vi "ECDChromBetrachterPC.vi"() -> ()   [LabVIEW 2010]
panel:
  in  "Zyklus":i32 min=0 max=385 step=1
  in  "Methode":i32 min=0 max=0 step=1
  out "Name":string
  in  "Beenden":bool
  out "Chrom":cluster{dbl, dbl}[](graph)
  in  "anzeigen":bool
  in  "Pfad":path
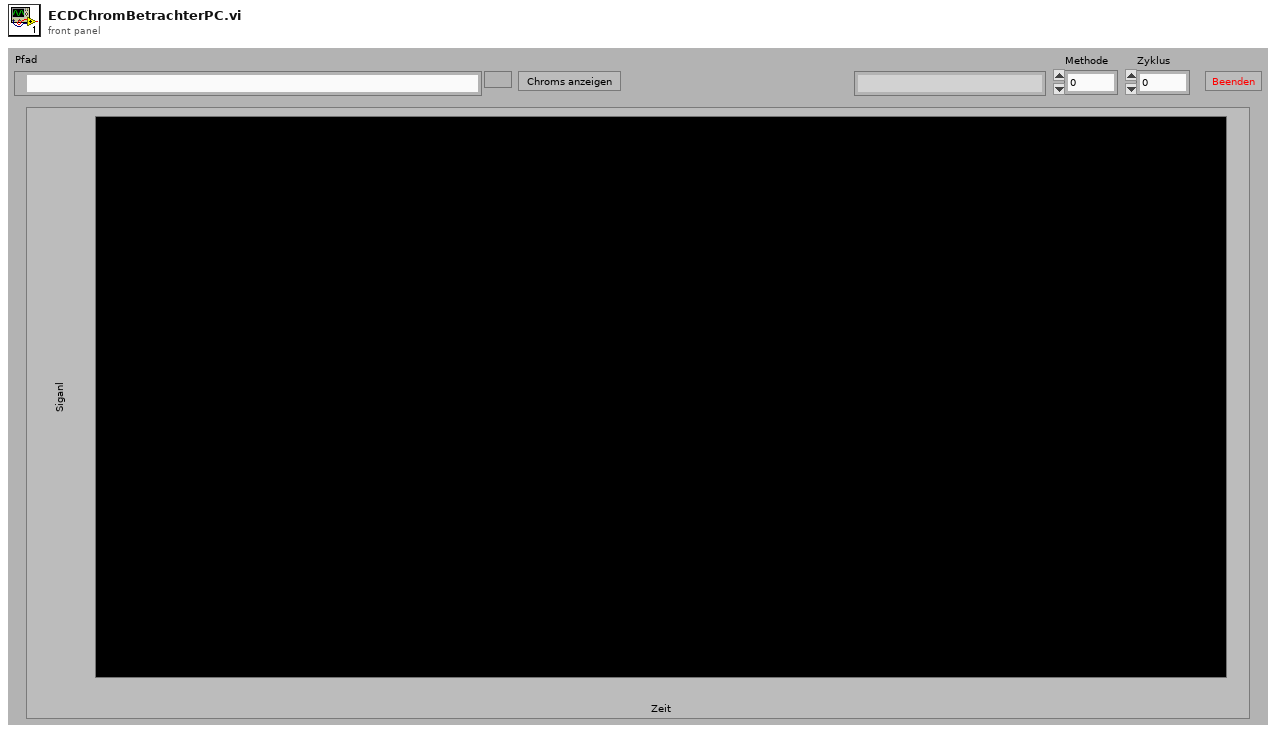
[diagram p1: front panel]
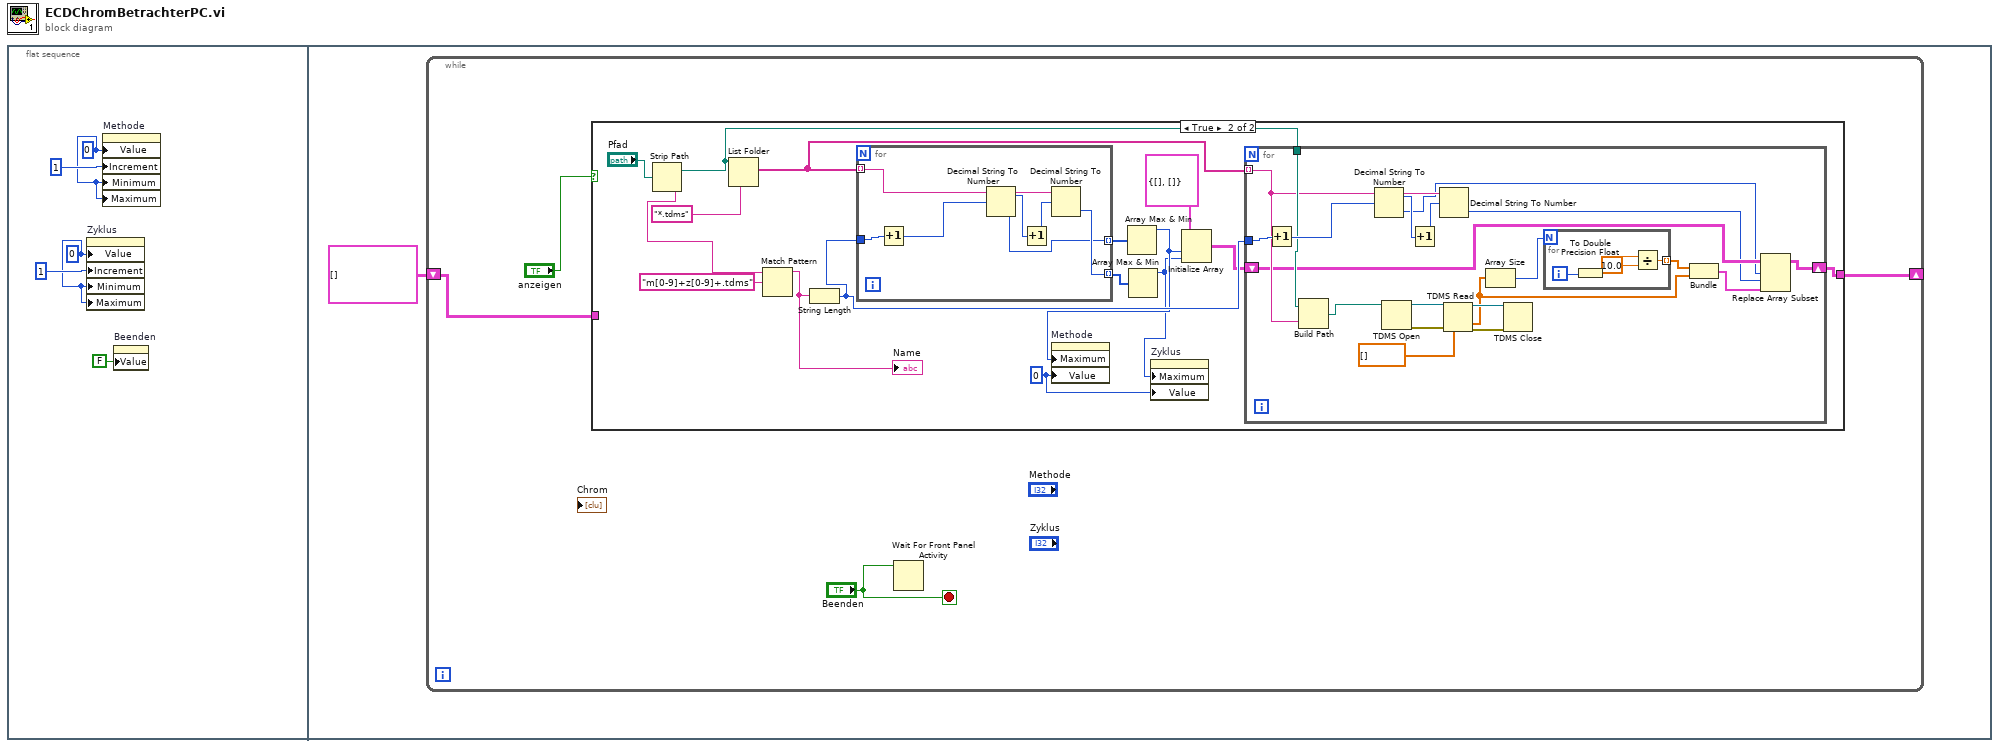
[diagram p0: block diagram]
diagram:
  n1 = flat-sequence {
    frame #0 {
      w2 = 0 ("Methode")
      w4 = 0 ("Methode")
      n2 = property on="Zyklus" class="DigWert (strikt)"("Value"=w2, "Increment"=1, "Minimum"=w2, "Maximum"=w2) -> ()  [unwired: 2 in, 2 out]
      n3 = property on="Methode" class="DigWert (strikt)"("Value"=w4, "Increment"=1, "Minimum"=w4, "Maximum"=w4) -> ()  [unwired: 2 in, 2 out]
      n4 = property on="Beenden" class="Bool. (strikt)"("Value"=FALSE ("Beenden")) -> ()  [unwired: 2 in, 2 out]
    }
    frame #1 {
      n5 = while {
        shift-right: [w8] -> _
        shift-left: cluster{dbl[], dbl[]}[][] [] -> [w7]
        stop <- "Beenden" stop-if-true
        n6 = case shown="True" "anzeigen" {
          tunnel: [w11 w15] -> w8
          tunnel: w7 -> [w11 _]
          frame False {
          }
          frame True {
            w12 = 0 ("Methode")
            n7 = Strip Path(path="Pfad") -> (stripped path=w17:path, name=w25:string)
            n8 = List Folder(path=w17, pattern="*.tdms" ("Muster")) -> (filenames=w18:string[])  [unwired: 2 in, 3 out]
            n9 = Match Pattern(string=w25, regular expression="m[0-9]+z[0-9]+.tdms" ("Regulärer Ausdruck")) -> (before substring=w23:string)  [unwired: 1 in, 3 out]
            "Name" <- w23
            n10 = String Length(string=w23) -> (length=w19:i32)
            n11 = for {
              tunnel: w18 -> [w54] mode=indexing
              tunnel: w19 -> [w56]
              tunnel: [w53] -> w21 mode=indexing
              tunnel: [w52] -> w22 mode=indexing
              n12 = Increment(x=w56) -> (x+1=w55:i32)
              n13 = Decimal String To Number(string=w54, offset=w55) -> (offset past number=w58:i32, number=w52:i32)  [unwired: 1 in]
              n14 = Increment(x=w58) -> (x+1=w57:i32)
              n15 = Decimal String To Number(string=w54, offset=w57) -> (number=w53:i32)  [unwired: 1 in, 1 out]
            }
            n16 = Array Max & Min(array=w22) -> (max value=w14:i32)  [unwired: 3 out]
            n17 = property on="Methode" class="DigWert (strikt)"("Maximum"=w14, "Value"=w12) -> ()  [unwired: 2 in, 2 out]
            n18 = Array Max & Min(array=w21) -> (max value=w13:i32)  [unwired: 3 out]
            n19 = property on="Zyklus" class="DigWert (strikt)"("Maximum"=w13, "Value"=w12) -> ()  [unwired: 2 in, 2 out]
            n20 = Initialize Array(cluster{dbl[], dbl[]} {[], []} ("Ausgangs-Cluster"), w14, w13) -> (w16:cluster{dbl[], dbl[]}[][])
            n21 = for {
              tunnel: w18 -> [w36] mode=indexing
              tunnel: w19 -> [w45]
              tunnel: w17 -> [w37]
              shift-right: [w28] -> w15
              shift-left: w16 -> [w32]
              n22 = Increment(x=w45) -> (x+1=w44:i32)
              n23 = Build Path(base path=w37, name or relative path=w36) -> (appended path=w43:path)
              n24 = Decimal String To Number(string=w36, offset=w44) -> (offset past number=w47:i32, number=w31:i32)  [unwired: 1 in]
              n25 = TDMS Open(11:w43) -> (0:w41:errorcluster, 3:w42:refnum<k34>)  [unwired: 5 in]
              n26 = Increment(x=w47) -> (x+1=w46:i32)
              n27 = Decimal String To Number(string=w36, offset=w46) -> (number=w30:i32)  [unwired: 1 in, 1 out]
              n28 = TDMS Read(0:w42, 11:w41, 12:dbl[] []) -> (4:w40:refnum<k34>, 10:w33:dbl[], 15:w39:errorcluster)  [unwired: 4 in, 3 out]
              n29 = Array Size(array=w33) -> (size(s)=w35:i32)
              n30 = TDMS Close(8:w39, 11:w40) -> ()  [unwired: 2 out]
              n31 = for {
                N: w35 -> [_]
                tunnel: [w48] -> w34 mode=indexing
                i -> [w51]
                n32 = To Double Precision Float(number=w51) -> (double precision float=w50:dbl)
                n33 = Divide(x=w50, y=10.0) -> (x/y=w48:dbl)
              }
              n34 = Bundle(w34, w33) -> (w29:cluster{dbl[], dbl[]})  [unwired: 1 in]
              n35 = Replace Array Subset(array=w32, new element=w29, index (row)=w31, index (col)=w30) -> (w28:cluster{dbl[], dbl[]}[][])
            }
          }
        }
        n36 = Wait For Front Panel Activity(3:"Beenden") -> ()  [unwired: 2 in, 1 out]
      }
    }
  }
